vi "_PC_Spectrafilter get_new_group_name.vi"(1 "spectra filter param out":T1) -> (0 "new group name":string)   [LabVIEW 2018]
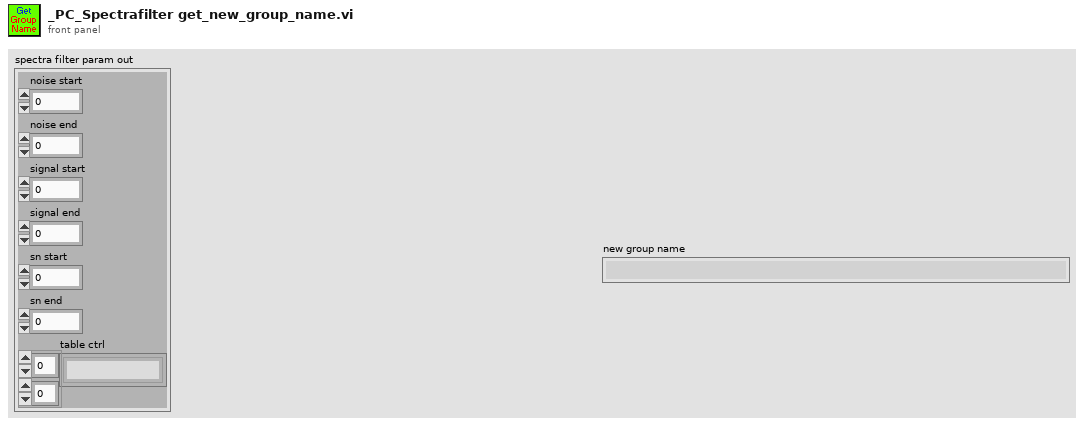
[diagram p1: front panel]
types:
  T1 = cluster{"noise start":dbl, "noise end":dbl, "signal start":dbl, "signal end":dbl, "sn start":dbl, "sn end":dbl, "table ctrl":string[][]}
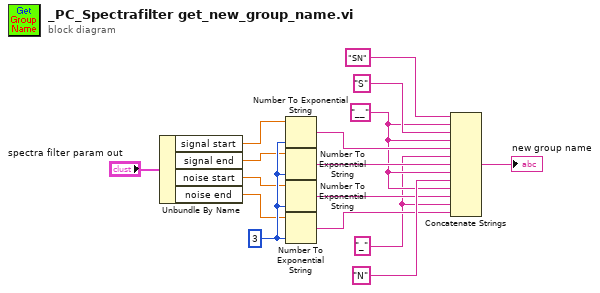
[diagram p0: block diagram]
diagram:
  w1 = "_"
  w15 = i16 3 ("precision (6)")
  w4 = "__"
  n1 = Unbundle By Name("spectra filter param out") -> ("signal start"=w14:dbl, "signal end"=w13:dbl, "noise start"=w12:dbl, "noise end"=w11:dbl)
  n2 = Number To Exponential String(number=w14, precision (6)=w15) -> (E-format string=w8:string)  [unwired: 2 in]
  n3 = Number To Exponential String(number=w13, precision (6)=w15) -> (E-format string=w6:string)  [unwired: 2 in]
  n4 = Number To Exponential String(number=w12, precision (6)=w15) -> (E-format string=w3:string)  [unwired: 2 in]
  n5 = Number To Exponential String(number=w11, precision (6)=w15) -> (E-format string=w2:string)  [unwired: 2 in]
  n6 = Concatenate Strings("SN", w4, "S", w4, w8, w1, w6, w4, "N", w4, w3, w1, w2) -> (→"new group name":string)
